vi "Formula NOede.vi"() -> ()   [LabVIEW 2011]
panel:
  out "z":dbl
  out "y":dbl
  in  "d":dbl
  in  "c":dbl
  in  "b":dbl
  in  "a":dbl
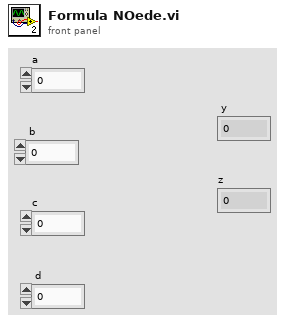
[diagram p1: front panel]
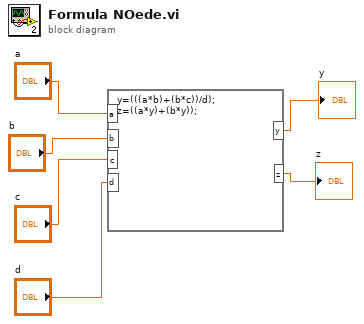
[diagram p0: block diagram]
diagram:
  n1 = formula code="y=(((a*b)+(b*c))/d);\nz=((a*y)+(b*y));"("a"="a", "b"="b", "c"="c", "d"="d") -> ("y"=→"y":dbl, "z"=→"z":dbl)
